vi "Operation.vi"(0 "Add in":refnum<class "Add.lvclass">, 11 "Error In":errorcluster) -> (4 "Add out":refnum<class "Add.lvclass">, 15 "Error Out":errorcluster)   [LabVIEW 2020, in "Add.lvclass"]
doc: "This Method is to add two numbers."
uses:
  Add.lvclass
  Add.lvclass/Add.ctl
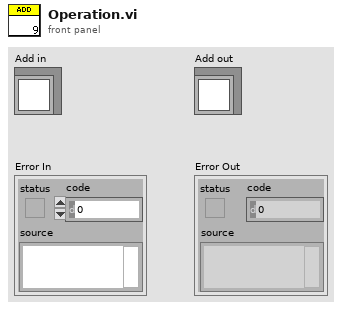
[diagram p1: front panel]
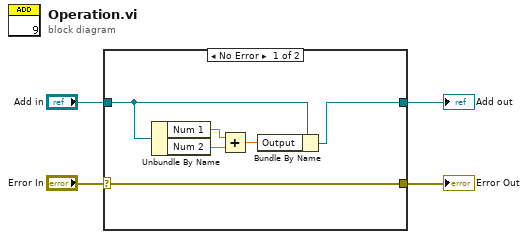
[diagram p0: block diagram]
diagram:
  n1 = case shown="No Error" "Error In" {
    selector: "Error In" -> [w10 w12]
    tunnel: [w10 w12] -> w3
    tunnel: [w9 w11] -> w1
    tunnel: "Add in" -> [w8 w11]
    frame No Error {
      n2 = Unbundle By Name(w8) -> ("Num 1"=w6:dbl, "Num 2"=w7:dbl)
      n3 = Add(x=w6, y=w7) -> (x+y=w5:dbl)
      n4 = Bundle By Name(cluster=w8, "Output"=w5) -> (w9:refnum<class "Add.lvclass">)
    }
    frame Error {
    }
  }
  "Error Out" <- w3
  "Add out" <- w1
